vi "TSM Relay Control Connections_v2.vi"(0 "TSM context in":T1, 5 "Relay/Action Connections":T4[](array[typedef]) {"Relay Action" items=["Open Relay"=20, "Close Relay"=21]}, 7 "Settling Time (s)":dbl, 11 "error in":errorcluster) -> (4 "TSM context out":T1, 8 "Completed Relay Operations":T2[](array[typedef]) {"Desired State" items=["Open Relay"=20, "Close Relay"=21]}, 15 "error out":errorcluster)   [LabVIEW 2019]
doc: "Performs actions on the corresponding Relays as specified by the Relay Connections input array, where each element in the array corresponds to a unique Relay and action pair."
uses:
  Pin Map/TSM Relay to Action Map.ctl
  <vilib>/NI_TestStand_SemiconductorModule/NI_TestStand_Semiconductor_Module.lvlibp/1abvi3w/instr.lib/niSwitch/niswitch.llb/niSwitch Relay Action.ctl
  <vilib>/NI_TestStand_SemiconductorModule/NI_TestStand_Semiconductor_Module.lvlibp/PinMap/General/SemiconductorModuleContext.ctl
  SubVIs/TSM Relay Completed Operations.ctl
  <instrlib>/niSwitch/niSwitch.llb/niSwitch Relay Action.ctl
  SSC/SSC Relay Control Core.vi
  SSC/Single SSC Relay NI-Switch Control.vi
  SSC/Single SSC Relay Fill Additional Error info.vi
  SSC/SSC Relay Expand Action Array to All Sessions.vi
  <vilib>/Utility/error.llb/Error Cluster From Error Code.vi
  <instrlib>/niSwitch/niSwitch.llb/niSwitch Get Relay Position.vi
  <instrlib>/niSwitch/niSwitch.llb/niSwitch Relay Control.vi
  <vilib>/Utility/High Resolution Polling Wait.vi
  <vilib>/NI_TestStand_SemiconductorModule/NI_TestStand_Semiconductor_Module.lvlibp
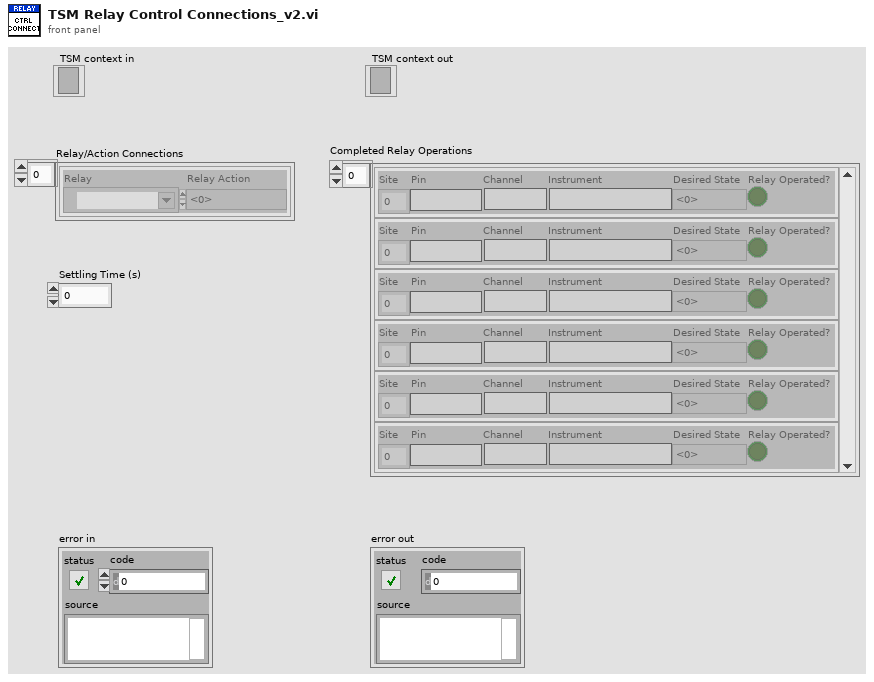
[diagram p1: front panel]
types:
  T1 = typedef "NI_TestStand_Semiconductor_Module.lvlibp/SemiconductorModuleContext.ctl" = refnum<k7>
  T2 = typedef "TSM Relay Completed Operations.ctl" = cluster{"Site":i32, "Pin":string, "Channel":string, "Instrument":string, "Desired State":T3, "Relay Operated?":bool}
  T3 = typedef "niSwitch Relay Action.ctl" = i32
  T4 = typedef "TSM Relay to Action Map.ctl" = cluster{"Relay":tag, "Relay Action":T5}
  T5 = typedef "NI_TestStand_Semiconductor_Module.lvlibp/niSwitch Relay Action.ctl" = i32
  T6 = typedef "TSM Relay Config.ctl" = cluster{"SSC Relay with Action":cluster{"SSC Relay":T7, "Relay Action":T3}[], "Pins":string[], "TSM Site Numbers":i32[], "Pin Query Context":refnum<class "MultiplePinMultipleSessionQueryContext.lvclass">}
  T7 = typedef "SSC Relay.ctl" = cluster{"Relay":string, "Site":i32, "Session":refnum<k15>, "Channel":string}
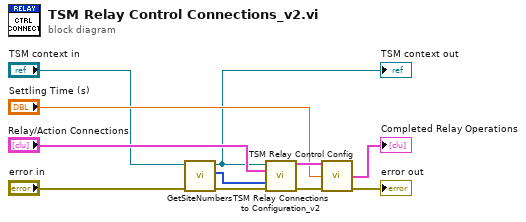
[diagram p0: block diagram]
diagram:
  n1 = call <vilib>:"GetSiteNumbers.vi"("error in (no error)"="error in", "Semiconductor Module Context"="TSM context in") -> ("error out"=w4:errorcluster, "Site Numbers"=w1:i32[], "Semiconductor Module Context Out"=w2:T1)  [unwired: 6 in, 1 out]
  "TSM context out" <- w2
  n2 = call "TSM Relay Connections to Configuration_v2.vi"("TSM Context"=w2, "Relay/Action Connections"="Relay/Action Connections", "TSM Site Numbers"=w1, "error in"=w4) -> ("TSM Relay Configuration"=w8:T6, "error out"=w9:errorcluster)  [unwired: 10 in]
  n3 = call "TSM Relay Control Config.vi"("TSM Relay Configuration in"=w8, "Settling Time (s)"="Settling Time (s)", "error in"=w9) -> ("Completed Relay Operations"=→"Completed Relay Operations":T2[], "error out"=→"error out":errorcluster)  [unwired: 10 in, 1 out]
